vi "Place_picture_on_graph.vi"(0 "ImgArray":refnum<vi>) -> (1 "GraphPosition":cluster{i32, i32}, 2 "PlotAreaSize":cluster{i32, i32}, 3 "PicturePosition":cluster{i32, i32}, 4 "DrawAreaSize":cluster{u32, u32})   [LabVIEW 2011]
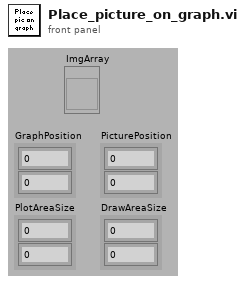
[diagram p1: front panel]
types:
  T1 = typedef "LVBoundsTypeDef.ctl" = cluster{"Width":u32, "Height":u32}
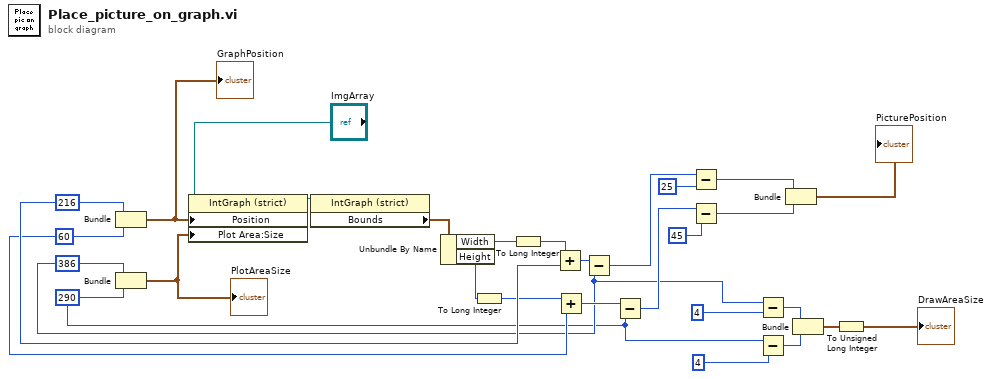
[diagram p0: block diagram]
diagram:
  w8 = 290
  w9 = 386
  w24 = 60
  w26 = 216
  n1 = Bundle(w26, w24) -> (w28:cluster{i32, i32})  [unwired: 1 in]
  "GraphPosition" <- w28
  n2 = Bundle(w9, w8) -> (w27:cluster{i32, i32})  [unwired: 1 in]
  "PlotAreaSize" <- w27
  n3 = property class="IntGraph (strict)"(reference="ImgArray", "Position"=w28, "Plot Area:Size"=w27) -> (reference out=w1:refnum<vi>)  [unwired: 1 in, 1 out]
  n4 = property class="IntGraph (strict)"(reference=w1) -> ("Bounds"=w12:T1)  [unwired: 1 in, 2 out]
  n5 = Unbundle By Name(w12) -> ("Width"=w22:u32, "Height"=w25:u32)
  n6 = To Long Integer(number=w25) -> (32bit integer=w23:i32)
  n7 = To Long Integer(number=w22) -> (32bit integer=w21:i32)
  n8 = Add(x=w21, y=w26) -> (x+y=w19:i32)
  n9 = Add(x=w23, y=w24) -> (x+y=w20:i32)
  n10 = Subtract(x=w19, y=w9) -> (x-y=w18:i32)
  n11 = Subtract(x=w20, y=w8) -> (x-y=w17:i32)
  n12 = Subtract(x=w18, y=25) -> (x-y=w15:i32)
  n13 = Subtract(x=w17, y=45) -> (x-y=w16:i32)
  n14 = Subtract(x=w9, y=4) -> (x-y=w10:i32)
  n15 = Subtract(x=w8, y=4) -> (x-y=w11:i32)
  n16 = Bundle(w15, w16) -> (→"PicturePosition":cluster{i32, i32})  [unwired: 1 in]
  n17 = Bundle(w10, w11) -> (w4:cluster{i32, i32})  [unwired: 1 in]
  n18 = To Unsigned Long Integer(number=w4) -> (unsigned 32bit integer=→"DrawAreaSize":cluster{u32, u32})
